vi "Open Dynamixel Port.vi"(8 "dynamixel_id":u8=1, 11 "Com port":refnum<visa-resource-name> caption="instrument handle") -> (0 "error out":errorcluster, 2 "Model Number":u32, 3 "port_num":i32)   [LabVIEW 2022 SP3]
uses:
  Dynamixel Global.vi
  Library/dxl.lvlib
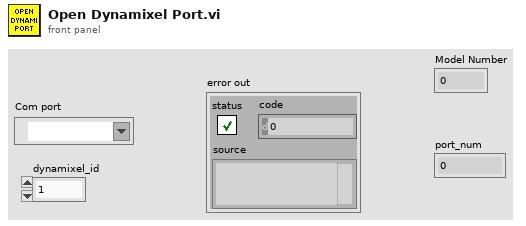
[diagram p1: front panel]
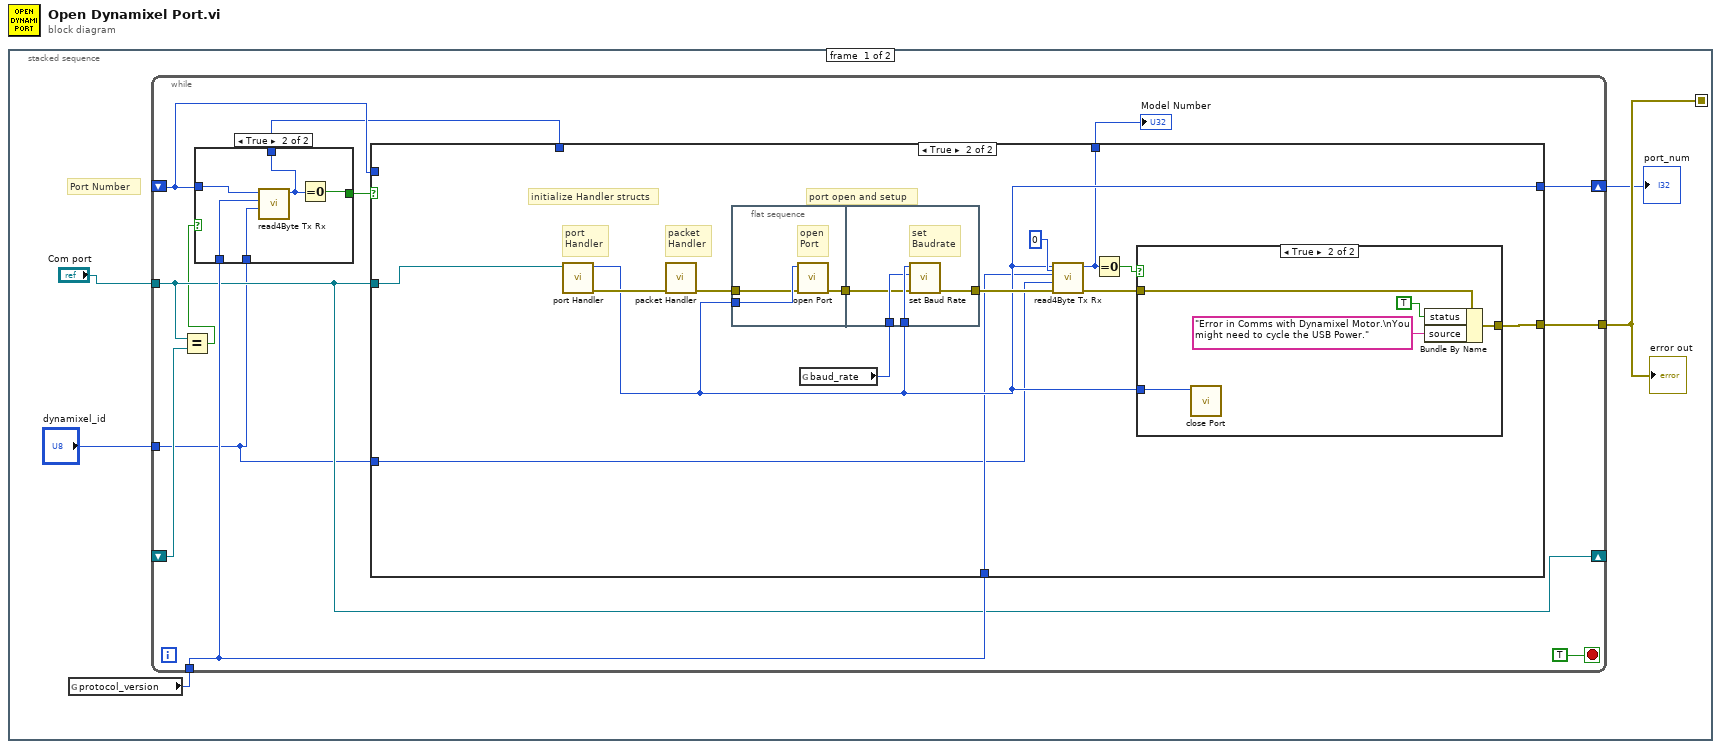
[diagram p0: block diagram]
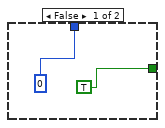
[diagram p2: hidden frame]
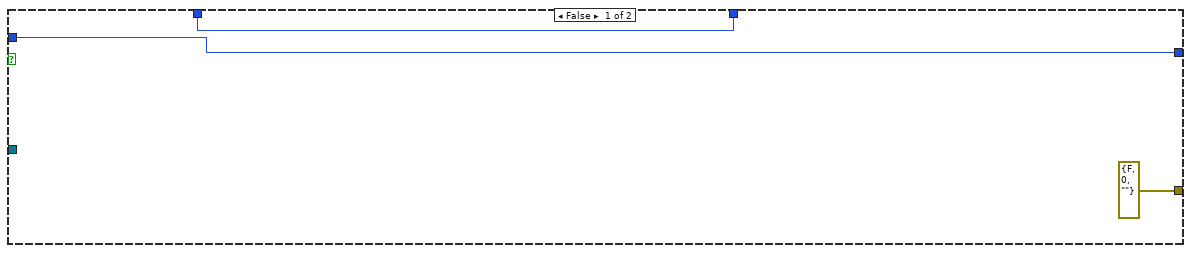
[diagram p3: hidden frame]
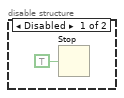
[diagram p7: hidden frame]
diagram:
  n1 = stacked-sequence {
    seq-local: [w5 _] -> [_ w55]
    frame #0 {
      # "Port Number"
      n2 = global read "Dynamixel Global.vi" "protocol_version"() -> (w4:i32)
      n3 = while {
        tunnel: [w17] -> w5
        shift-right: [w12] -> _
        shift-left: _ -> [w13]
        shift-right: [w16] -> w1
        shift-left: _ -> [w10]
        tunnel: w4 -> [w15]
        tunnel: "Com port" -> [w12]
        tunnel: "dynamixel_id" -> [w6]
        stop <- TRUE stop-if-true
        n4 = Equal?(x=w12, y=w13) -> (x = y?=w11:bool)
        n5 = case shown="True" w11 {
          tunnel: w15 -> [_ w24]
          tunnel: [TRUE w22] -> w14
          tunnel: w10 -> [_ w23]
          tunnel: [u32 0 ("function return") w21] -> w7
          tunnel: w6 -> [_ w20]
          frame False {
          }
          frame True {
            n6 = call "read4Byte Tx Rx.vi"("id"=w20, "protocol_version"=w24, "port_num"=w23) -> ("function return"=w21:u32)  [unwired: 7 in, 1 out]
            n7 = Equal To 0?(x=w21) -> (x = 0?=w22:bool)
          }
        }
        n8 = case shown="True" w14 {
          tunnel: [errorcluster {"status"=FALSE, "code"=0, "source"=""} ("error out") w33] -> w17
          tunnel: [w27 w32] -> w16
          tunnel: w15 -> [_ w31]
          tunnel: w10 -> [w27 _]
          tunnel: w12 -> [_ w30]
          tunnel: [w25 w29] -> w8
          tunnel: w7 -> [w25 _]
          tunnel: w6 -> [_ w28]
          frame False {
          }
          frame True {
            # "packet\nHandler"
            # "port\nHandler"
            # "port open and setup"
            # "initialize Handler structs"
            n9 = call "port Handler.vi"("port_name"=w30) -> ("error out"=w41:errorcluster, "function return"=w32:i32)  [unwired: 9 in]
            n10 = call "packet Handler.vi"("error in (no error)"=w41) -> ("error out"=w39:errorcluster)  [unwired: 10 in]
            n11 = flat-sequence {
              tunnel: w32 -> [w50]
              tunnel: w39 -> [w49]
              tunnel: [w48] -> w40
              tunnel: w32 -> [w54]
              tunnel: w38 -> [w53]
              tunnel: w40 -> [w52]
              tunnel: [w51] -> w36
              frame #0 {
                # "open\nPort"
                n12 = call "open Port.vi"("error in (no error)"=w49, "port_num"=w50) -> ("error out"=w48:errorcluster)  [unwired: 8 in, 1 out]
              }
              frame #1 {
                # "set\nBaudrate"
                n13 = call "set Baud Rate.vi"("error in (no error)"=w52, "baudrate"=w53, "port_num"=w54) -> ("error out"=w51:errorcluster)  [unwired: 7 in, 1 out]
              }
            }
            n14 = global read "Dynamixel Global.vi" "baud_rate"() -> (w38:i32)
            n15 = call "read4Byte Tx Rx.vi"("address"=u16 0, "error in (no error)"=w36, "id"=w28, "protocol_version"=w31, "port_num"=w32) -> ("error out"=w34:errorcluster, "function return"=w29:u32)  [unwired: 5 in]
            n16 = Equal To 0?(x=w29) -> (x = 0?=w35:bool)
            n17 = case shown="True" w35 {
              tunnel: w32 -> [_ w47]
              tunnel: w34 -> [w42 w46]
              tunnel: [w42 w43] -> w33
              frame False {
              }
              frame True {
                n18 = call "close Port.vi"("port_num"=w47) -> ()  [unwired: 10 in, 1 out]
                n19 = Bundle By Name(cluster=w46, "status"=TRUE, "source"="Error in Comms with Dynamixel Motor.\nYou might need to cycle the USB Power.") -> (w43:errorcluster)
              }
            }
          }
        }
        "Model Number" <- w8
      }
      "error out" <- w5
      "port_num" <- w1
    }
    frame #1 {
      n20 = case shown="Error .." w55 {
        frame No Error {
        }
        frame Error {
          n21 = disable-structure shown="Enabled" {
            frame Disabled {
              n22 = Stop(stop? (T)=TRUE) -> ()
            }
            frame Enabled {
            }
          }
        }
      }
    }
  }
